vi "Local Configuration.DMADPR0.Transfer Direction.Set.vi"(8 "error in (no error)":errorcluster, 10 "Transfer Direction":enum16{"Write", "Read"}(ring), 11 "GE 5565PIORC":refnum<class "GE 5565PIORC.lvclass">) -> (0 "error out":errorcluster, 3 "GE 5565PIORC out":refnum<class "GE 5565PIORC.lvclass">)   [LabVIEW 2016, in "GE 5565PIORC.lvclass"]
uses:
  GE 5565PIORC.lvclass
  Controls/Registers.Local Configuration.ctl
  GE 5565PIORC.lvclass/GE 5565PIORC.ctl
  <vilib>/Instr/_visa.llb/VISA Register Access Address Space.ctl
  Binary Operations/Set Bits U32.vi
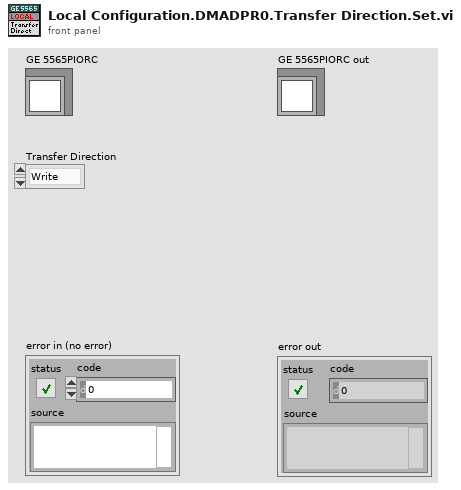
[diagram p1: front panel]
types:
  T1 = typedef "GE 5565PIORC.lvclass/Registers.Local Configuration.ctl" = enum16{"DMA Arbitration", "Interrupt Control and Status", "DMA Mode", "DMA PCI Address", "DMA Local Address", "DMA Transfer Size", "DMA Descriptor Pointer", "DMA Command/Status", "DMA PCI DAC Upper Address", "PCI PIO Address Range", "PCI PIO Base Address (Remap)"}
  T2 = typedef "VISA Register Access Address Space.ctl" = u16
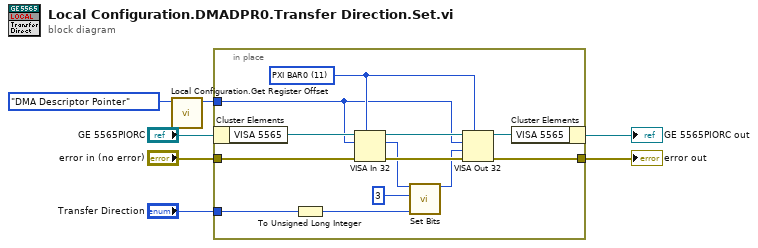
[diagram p0: block diagram]
diagram:
  n1 = call "Local Configuration.Get Register Offset.vi"("Local Configuration Register"=Registers.Local_Configuration."DMA Descriptor Pointer" ("Local Configration Register Offset")) -> ("Offset"=w1:u32)  [unwired: 10 in]
  n2 = in-place {
    in-place-border: "error in (no error)" -> [w19]
    in-place-border: [w15] -> w5
    in-place-border: "Transfer Direction" -> [w9]
    in-place-border: w1 -> [w8]
    w12 = T2 11 items=["VXI/VME A16"=1, "VXI/VME A24"=2, "VXI/VME A32"=3, "VXI/VME A64"=4, "PXI Memory Allocations"=9, "PXI Configuration"=10, "PXI BAR0"=11, "PXI BAR1"=12, "PXI BAR2"=13, "PXI BAR3"=14, "PXI BAR4"=15, "PXI BAR5"=16] ("Address Space")
    n3 = in-place-cluster #1("GE 5565PIORC") -> ("VISA 5565"=w20:refnum<visa-resource-name>)
    n4 = To Unsigned Long Integer(number=w9) -> (unsigned 32bit integer=w10:u32)
    n5 = VISA In 32(7:w12, 8:w19, 10:w8, 11:w20) -> (0:w17:errorcluster, 2:w13:u32, 3:w18:refnum<visa-resource-name>)
    n6 = call-poly "Set Bits.vi"("Value (0)"=w10, "Start Index (0)"=u8 3, "Register in"=w13) -> ("Register out"=w14:u32)  [unwired: 6 in, 2 out]
    n7 = VISA Out 32(7:w12, 8:w17, 9:w14, 10:w8, 11:w18) -> (0:w15:errorcluster, 3:w16:refnum<visa-resource-name>)
    n8 = in-place-cluster #1("VISA 5565"=w16) -> (→"GE 5565PIORC out":refnum<class "GE 5565PIORC.lvclass">)
  }
  "error out" <- w5
